vi "Update Non-SD Channels.vi"(7 "Type":T2, 8 "error in (no error)":errorcluster, 9 "Channel Names":string[](array[string]), 10 "Node Ptr In":T1 format="%.0x", 11 "SD Module in":refnum<class "SD Module.lvclass">) -> (0 "error out":errorcluster, 2 "Node Ptr Out":T1 format="%.0x", 3 "SD Module out":refnum<class "SD Module.lvclass">)   [LabVIEW 2019, in "Modules.lvlib" / "SD Module.lvclass"]
uses:
  SD Module.lvclass
  <vilib>/NI VeriStand/Custom Device API/Custom Device Channel Type.ctl
  <vilib>/NI VeriStand/Custom Device API/Custom Device Item Ref.ctl
  <vilib>/NI VeriStand/Custom Device API/Custom Device API.lvlib
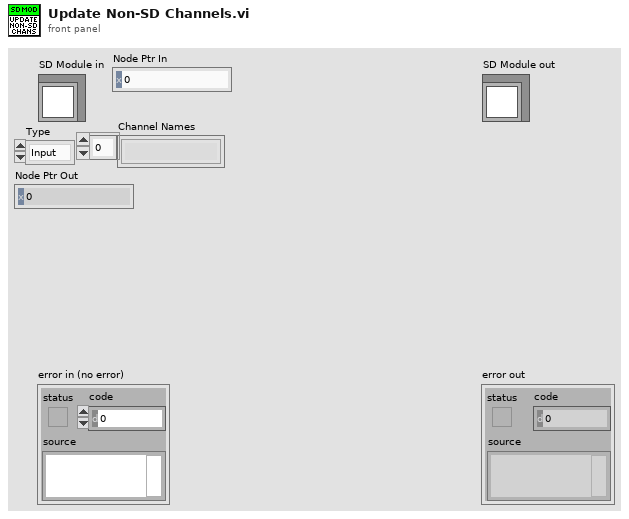
[diagram p1: front panel]
types:
  T1 = typedef "Custom Device API.lvlib/Custom Device Item Ref.ctl" = u64
  T2 = typedef "Custom Device API.lvlib/Custom Device Channel Type.ctl" = enum16{"Input", "Output"}
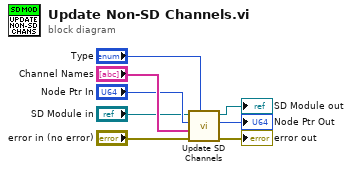
[diagram p0: block diagram]
diagram:
  n1 = call "Update SD Channels.vi"("Type"="Type", "error in (no error)"="error in (no error)", "Channel Names"="Channel Names", "Node Ptr In"="Node Ptr In", "SD Module in"="SD Module in") -> ("error out"=→"error out":errorcluster, "Node Ptr Out"=→"Node Ptr Out":T1, "SD Module out"=→"SD Module out":refnum<class "SD Module.lvclass">)  [unwired: 4 in]
